vi "ClimbWeight.vi"   [LabVIEW 2013]
uses:
  State_Machine_Enum.ctl
  <vilib>/Rock Robotics/WPI/Solenoid/WPI_SolenoidValue.ctl
  RefnameEnum.ctl
  Robot Global Data.vi
  <vilib>/Rock Robotics/WPI/Solenoid/WPI_SolenoidSetEnum.vi
types:
  T1 = typedef "State_Machine_Enum.ctl" = enum16{"Idle", "Start", "Do", "Stop", "Init"}
  T2 = typedef "WPI_SolenoidValue.ctl" = enum16{"Off", "On", "Forward", "Reverse"}
  T3 = typedef "RefnameEnum.ctl" = enum16{"FireLauncher", "Climber", "Shield", "TankDrive", "DriveEncoderL", "DriveEncoderR", "LauncherMotorRPM", "LauncherEncoderAnalog", "LauncherEncoderRPM", "ShooterLS", "DriveAlignLSLeft", "DriveAlignLSRight", "ClimbingLS", "LauncherEncoderAngle", "LauncherMotorAngle", "Gamepad1", "Gamepad2", "Compressor", "ClimbWeightSol3", "ClimbWeightSol4"}
  T4 = typedef "WPI_SolenoidDevRef.ctl" = cluster{"DevStatus":errorcluster, "Solenoid Module":T5, "Forward Solenoid Channel":T6, "Reverse Solenoid Channel":T6}
  T5 = typedef "FPGA_TypedefSolenoidModule.ctl" = enum16{"Solenoid Module 1", "Solenoid Module 2"}
  T6 = typedef "WPI_SolenoidChannel.ctl" = enum8{"Solenoid 1", "Solenoid 2", "Solenoid 3", "Solenoid 4", "Solenoid 5", "Solenoid 6", "Solenoid 7", "Solenoid 8", "Invalid"}
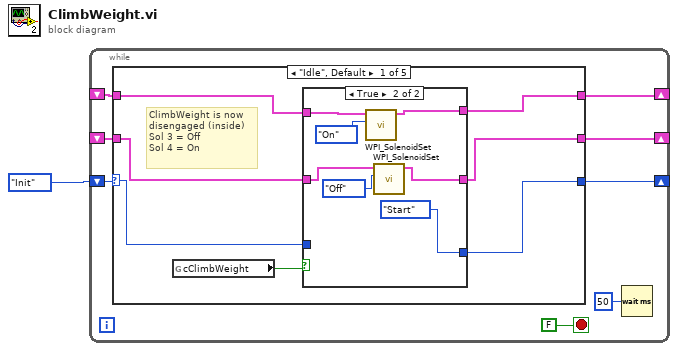
[diagram p0: block diagram]
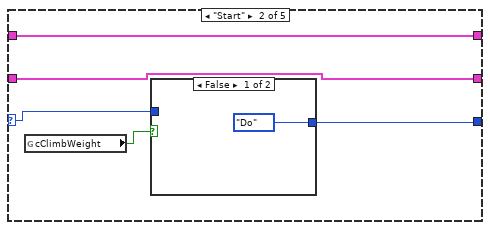
[diagram p3: hidden frame]
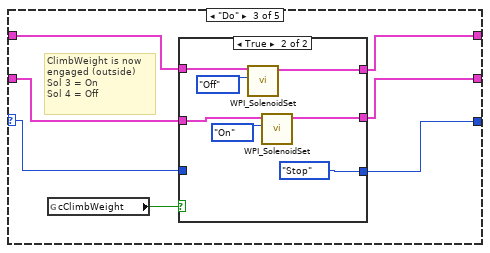
[diagram p5: hidden frame]
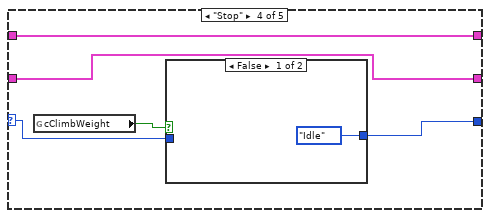
[diagram p7: hidden frame]
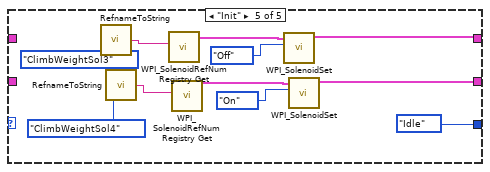
[diagram p9: hidden frame]
diagram:
  n1 = while {
    shift-right: [w8] -> _
    shift-left: State_Machine_Enum."Init" ("State") -> [w9]
    shift-right: [w7] -> _
    shift-left: _ -> [w6]
    shift-right: [w3] -> _
    shift-left: _ -> [w2]
    stop <- FALSE stop-if-true
    n2 = case shown="\"Idle\", Default" w9 {
      selector: w9 -> [w12 w28 w36 w53 _]
      tunnel: [w13 w29 w37 w54 State_Machine_Enum."Idle" ("State")] -> w8
      tunnel: [w14 w31 w38 w52 w66] -> w7
      tunnel: w6 -> [w15 w31 w39 w52 _]
      tunnel: [w10 w27 w34 w51 w58] -> w3
      tunnel: w2 -> [w11 w27 w35 w51 _]
      frame "Idle", Default {
        # "ClimbWeight is now\ndisengaged (inside)\nSol 3 = Off\nSol 4 = On"
        n3 = global read "Robot Global Data.vi" "cClimbWeight"() -> (w16:bool)
        n4 = case shown="True" w16 {
          tunnel: w15 -> [w18 w26]
          tunnel: [w18 w25] -> w14
          tunnel: [w19 State_Machine_Enum."Start" ("State")] -> w13
          tunnel: w12 -> [w19 _]
          tunnel: w11 -> [w17 w21]
          tunnel: [w17 w20] -> w10
          frame False {
          }
          frame True {
            n5 = call-poly <vilib>:"WPI_SolenoidSet.vi"("Value"=WPI_SolenoidValue."On", "SolenoidDevRef"=w26) -> ("SolenoidDevRef"=w25:T4)  [unwired: 8 in, 1 out]
            n6 = call-poly <vilib>:"WPI_SolenoidSet.vi"("Value"=WPI_SolenoidValue."Off", "SolenoidDevRef"=w21) -> ("SolenoidDevRef"=w20:T4)  [unwired: 8 in, 1 out]
          }
        }
      }
      frame "Start" {
        n7 = global read "Robot Global Data.vi" "cClimbWeight"() -> (w30:bool)
        n8 = case shown="False" w30 {
          tunnel: [State_Machine_Enum."Do" ("State") w33] -> w29
          tunnel: w28 -> [_ w33]
          frame False {
          }
          frame True {
          }
        }
      }
      frame "Do" {
        # "ClimbWeight is now\nengaged (outside)\nSol 3 = On\nSol 4 = Off"
        n9 = global read "Robot Global Data.vi" "cClimbWeight"() -> (w40:bool)
        n10 = case shown="True" w40 {
          tunnel: w39 -> [w43 w50]
          tunnel: [w43 w49] -> w38
          tunnel: [w42 State_Machine_Enum."Stop" ("State")] -> w37
          tunnel: w36 -> [w42 _]
          tunnel: w35 -> [w41 w45]
          tunnel: [w41 w44] -> w34
          frame False {
          }
          frame True {
            n11 = call-poly <vilib>:"WPI_SolenoidSet.vi"("Value"=WPI_SolenoidValue."Off", "SolenoidDevRef"=w50) -> ("SolenoidDevRef"=w49:T4)  [unwired: 8 in, 1 out]
            n12 = call-poly <vilib>:"WPI_SolenoidSet.vi"("Value"=WPI_SolenoidValue."On", "SolenoidDevRef"=w45) -> ("SolenoidDevRef"=w44:T4)  [unwired: 8 in, 1 out]
          }
        }
      }
      frame "Stop" {
        n13 = global read "Robot Global Data.vi" "cClimbWeight"() -> (w55:bool)
        n14 = case shown="False" w55 {
          tunnel: [State_Machine_Enum."Idle" ("State") w57] -> w54
          tunnel: w53 -> [_ w57]
          frame False {
          }
          frame True {
          }
        }
      }
      frame "Init" {
        n15 = call "RefnameToString.vi"("Enum"=RefnameEnum."ClimbWeightSol3") -> ("Refname"=w63:string)
        n16 = call "RefnameToString.vi"("Enum"=RefnameEnum."ClimbWeightSol4") -> ("Refname"=w62:string)
        n17 = call <vilib>:"WPI_SolenoidRefNum Registry Get.vi"("refnum name"=w63) -> ("SolenoidDevRef"=w67:T4)  [unwired: 9 in, 1 out]
        n18 = call <vilib>:"WPI_SolenoidRefNum Registry Get.vi"("refnum name"=w62) -> ("SolenoidDevRef"=w59:T4)  [unwired: 9 in, 1 out]
        n19 = call-poly <vilib>:"WPI_SolenoidSet.vi"("Value"=WPI_SolenoidValue."Off", "SolenoidDevRef"=w67) -> ("SolenoidDevRef"=w66:T4)  [unwired: 8 in, 1 out]
        n20 = call-poly <vilib>:"WPI_SolenoidSet.vi"("Value"=WPI_SolenoidValue."On", "SolenoidDevRef"=w59) -> ("SolenoidDevRef"=w58:T4)  [unwired: 8 in, 1 out]
      }
    }
    n21 = Wait (ms)(milliseconds to wait=u32 50) -> ()  [unwired: 1 out]
  }
